vi "SubInitialize.vi"(7 "communication settings":T1={"deviceName"="EPOS4", "protocolStackName"="CANopen", "baudrate"=1000000}, 8 "error in (no error)":errorcluster, 9 "modes of operations":i8(ring)=1 items=["Profile Position Mode"=1, "Profile Velocity Mode"=3, "Homing Mode"=6, "Interpolated Position Mode"=7, "Position Mode"=-1, "Velocity Mode"=-2, "Current Mode"=-3, "Master Encoder Mode"=-5, "Step Direction Mode"=-6], 10 "nodeId":u16=2, 11 "axis in":cluster{"keyHandle":u32, "nodeId":u16}={"keyHandle"=0, "nodeId"=1}) -> (0 "error out":errorcluster, 3 "axis out":cluster{"keyHandle":u32, "nodeId":u16}={"keyHandle"=0, "nodeId"=1})   [LabVIEW 2018]
doc: "<B>Initialize</B> opens the port for sending and receiving commands. This function opens interfaces with the RS232 or USB and with CANopen boards.\nFor exact names use the functions <B>VCS Get Device Name Selection</B>, <B>VCS Get Protocol Stack Name Selection</B>, <B>VCS Get Interface Name Selection</B>, <B>VCS Get Port Name Selection</B> and <B>VCS Get Baudrate Selection</B>.\nThe function sets a new operational mode and clears all errors."
panel:
  # "(c) 2007 - 2017 maxon motor ag.  ALL RIGHTS RESERVED."
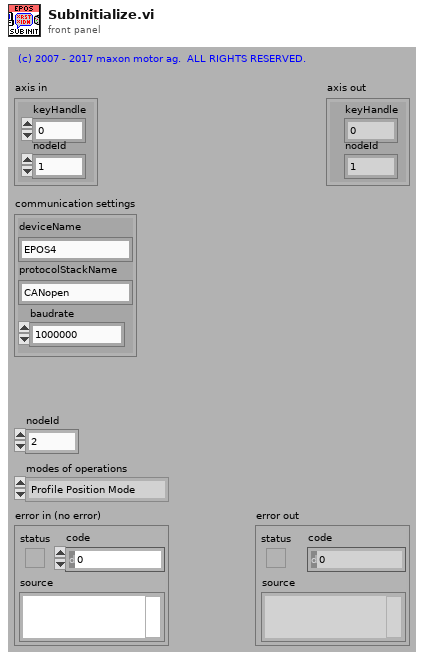
[diagram p1: front panel]
types:
  T1 = cluster{"deviceName":string, "protocolStackName":string, "baudrate":u32}
  T2 = cluster{"deviceName":string, "protocolStackName":string}
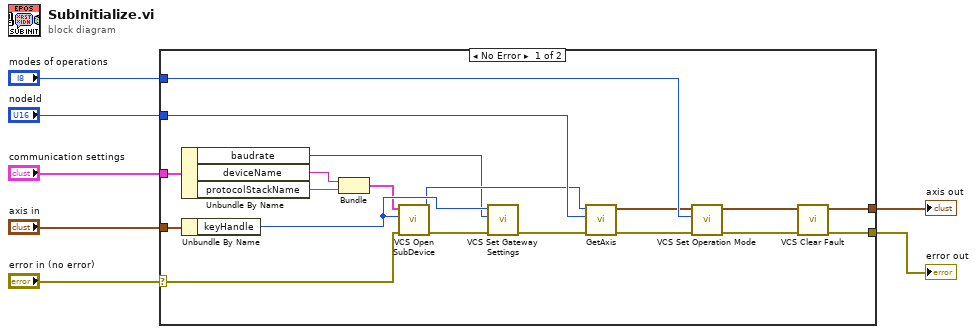
[diagram p0: block diagram]
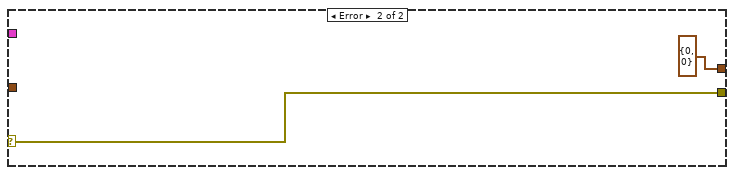
[diagram p2: hidden frame]
diagram:
  n1 = case shown="No Error" "error in (no error)" {
    selector: "error in (no error)" -> [w14 w28]
    tunnel: [w24 w28] -> w6
    tunnel: "nodeId" -> [w23 _]
    tunnel: "modes of operations" -> [w22 _]
    tunnel: [w19 cluster{"keyHandle":u32, "nodeId":u16} {"keyHandle"=0, "nodeId"=0} ("axis out")] -> w3
    tunnel: "communication settings" -> [w13 _]
    tunnel: "axis in" -> [w18 _]
    frame No Error {
      n2 = Unbundle By Name(w13) -> ("baudrate"=w8:u32, "deviceName"=w12:string, "protocolStackName"=w11:string)
      n3 = Unbundle By Name(w18) -> ("keyHandle"=w17:u32)
      n4 = Bundle("deviceName"=w12, "protocolStackName"=w11) -> (w10:T2)  [unwired: 1 in]
      n5 = call "VCS Open SubDevice.vi"("error in (no error)"=w14, "deviceHandle"=w17, "device in"=w10) -> ("error out"=w15:errorcluster, "keyHandle out"=w9:u32)  [unwired: 7 in]
      n6 = call "VCS Set Gateway Settings.vi"("error in (no error)"=w15, "Baudrate"=w8, "keyHandle in"=w17) -> ("error out"=w16:errorcluster)  [unwired: 7 in, 1 out]
      n7 = call "GetAxis.vi"("error in (no error)"=w16, "nodeId"=w23, "keyHandle in"=w9) -> ("error out"=w26:errorcluster, "axis out"=w21:cluster{"keyHandle":u32, "nodeId":u16})  [unwired: 7 in]
      n8 = call "VCS Set Operation Mode.vi"("error in (no error)"=w26, "modes of operations"=w22, "axis in"=w21) -> ("error out"=w25:errorcluster, "axis out"=w20:cluster{"keyHandle":u32, "nodeId":u16})  [unwired: 7 in]
      n9 = call "VCS Clear Fault.vi"("error in (no error)"=w25, "axis in"=w20) -> ("error out"=w24:errorcluster, "axis out"=w19:cluster{"keyHandle":u32, "nodeId":u16})  [unwired: 8 in]
    }
    frame Error {
    }
  }
  "error out" <- w6
  "axis out" <- w3
